vi "LensMotor_stop.vi"(7 "modIdTag":string="S1", 8 "error in (no error)":errorcluster, 11 "channel":refnum<k24>) -> (0 "error out":errorcluster)   [LabVIEW 2021]
uses:
  D:/psychometric_function_v2/lib/Grpc.Core.dll
  lib/Grpc.Core.dll
  D:/psychometric_function_v2/lib/FossilProtosSharp.dll
  lib/FossilProtosSharp.dll
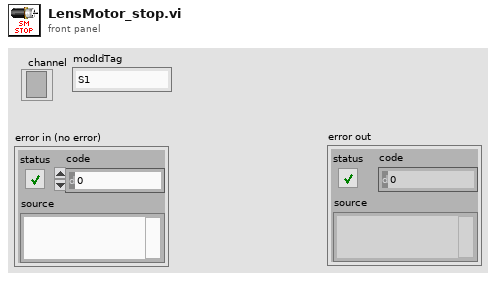
[diagram p1: front panel]
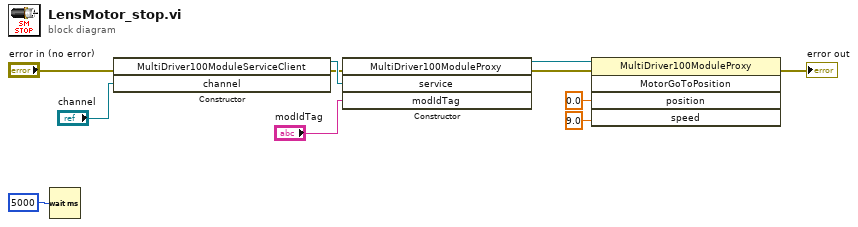
[diagram p0: block diagram]
diagram:
  n1 = Wait (ms)(milliseconds to wait=u32 5000) -> ()  [unwired: 1 out]
  n2 = constructor class="MultiDriver100ModuleServiceClie"(error in="error in (no error)", "channel"="channel") -> (reference out=w8:refnum<k24>, error out=w7:errorcluster)  [unwired: 2 in, 2 out]
  n3 = constructor class="MultiDriver100ModuleProxy"(error in=w7, "service"=w8, "modIdTag"="modIdTag") -> (reference out=w6:refnum<k24>, error out=w5:errorcluster)  [unwired: 2 in, 3 out]
  n4 = invoke class="MultiDriver100ModuleProxy" method="MotorGoToPosition"(reference=w6, error in=w5, "position"=sgl 0.0, "speed"=sgl 9.0) -> (error out=→"error out":errorcluster)  [unwired: 1 in, 4 out]
